vi "MDML_reset.vi"(8 "error in (no error)":errorcluster, 10 "connMeta 5":T1, 11 "Experiment ID":string) -> (0 "error out":errorcluster)   [LabVIEW 2018]
uses:
  Downloads/mqtt_lv2013_201708181938/mqtt_lv2013/mqtt Folder/src/class/mqtt/mqttTypedef/mqttConnectionMeta.ctl
  Downloads/mqtt_lv2013_201708181938/mqtt_lv2013/mqtt Folder/src/class/mqtt/mqttTypedef/mqttQOSlevel.ctl
  Downloads/mqtt_lv2013_201708181938/mqtt_lv2013/mqtt Folder/src/class/mqtt/mqtt.lvclass
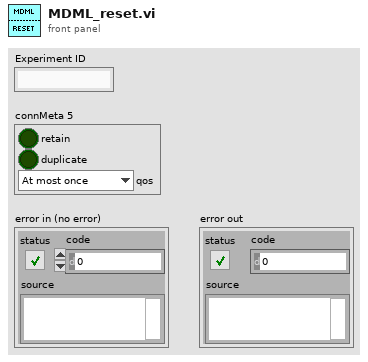
[diagram p1: front panel]
types:
  T1 = typedef "mqttConnectionMeta.ctl" = cluster{"retain":bool, "duplicate":bool, "qos":T2}
  T2 = typedef "mqttQOSlevel.ctl" = enum8{"At most once", "At least once", "Exactly once", "Reserved"}
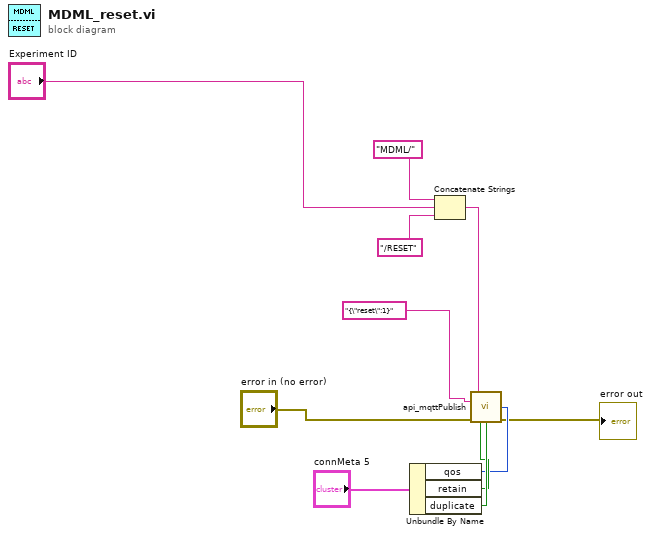
[diagram p0: block diagram]
diagram:
  n1 = Unbundle By Name("connMeta 5") -> ("qos"=w8:T2, "retain"=w9:bool, "duplicate"=w10:bool)
  n2 = Concatenate Strings("MDML/", "Experiment ID", "/RESET") -> (w5:string)
  n3 = call "api_mqttPublish.vi"("topic"=w5, "value"="{\"reset\":1}", "QoS (At most once)"=w8, "error in (no error)"="error in (no error)", "retain(F)"=w9, "duplicate(F)"=w10) -> ("error out"=→"error out":errorcluster)  [unwired: 8 in, 1 out]
